vi "UTIL Initialize Moving Average Temp.vi"(8 "Error In":errorcluster, 10 "element":dbl=22.0, 11 "Window Width":i32=10) -> (0 "Error Out":errorcluster, 3 "queue out":refnum<queue>)   [LabVIEW 2010]
doc: "Initialize a Moving Window Average routine by creating a fixed-length, Windows-sized Queue of Dbls, and initializing them to 0.\n\nInput:\n Window Size I32, default 10\n Error In\nOutput:\n Average Queue Fixed-length Queue of Dbl\n Error Out"
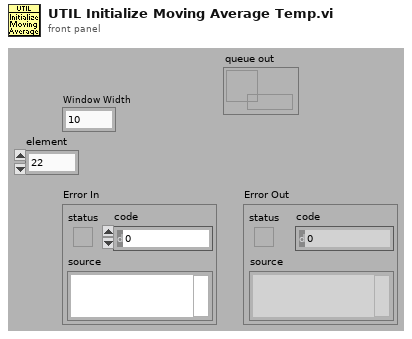
[diagram p1: front panel]
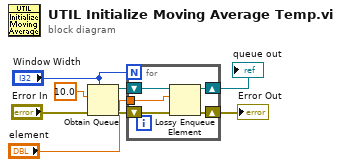
[diagram p0: block diagram]
diagram:
  n1 = Obtain Queue(max queue size (-1, unlimited)="Window Width", element data type=10.0 ("element"), error in (no error)="Error In") -> (queue out=w7:refnum<queue>, error out=w8:errorcluster)  [unwired: 2 in, 1 out]
  n2 = for {
    N: "Window Width" -> [_]
    shift-right: [w12] -> w5
    shift-left: w8 -> [w13]
    shift-right: [w10] -> w2
    shift-left: w7 -> [w11]
    tunnel: "element" -> [w9]
    n3 = Lossy Enqueue Element(queue=w11, element=w9, error in (no error)=w13) -> (queue out=w10:refnum<queue>, error out=w12:errorcluster)  [unwired: 2 out]
  }
  "Error Out" <- w5
  "queue out" <- w2
